vi "Graph Ref AE.vi"(7 "Action":enum16{"READ", "WRITE"}(ring), 10 "Graph Ref In":refnum<vi>[](array[refnum])) -> (2 "Graph Ref Out":refnum<vi>[](array[refnum]))   [LabVIEW 2014]
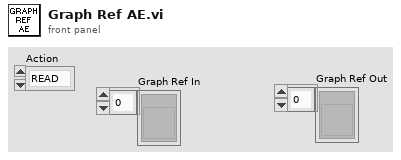
[diagram p1: front panel]
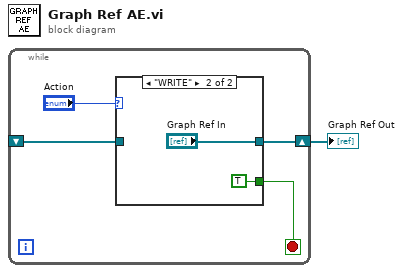
[diagram p0: block diagram]
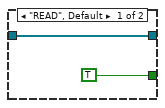
[diagram p2: hidden frame]
diagram:
  n1 = while {
    shift-right: [w5] -> w1
    shift-left: _ -> [w4]
    stop <- w2 stop-if-true
    n2 = case shown="\"WRITE\"" "Action" {
      tunnel: [w7 "Graph Ref In"] -> w5
      tunnel: w4 -> [w7 _]
      tunnel: [TRUE TRUE] -> w2
      frame "READ", Default {
      }
      frame "WRITE" {
      }
    }
  }
  "Graph Ref Out" <- w1
